vi "QuadRotor_Monitoring_LV2.vi"() -> ()   [LabVIEW 2015]
uses:
  <vilib>/Instr/_visa.llb/VISA Set IO Buffer Mask.ctl
  <vilib>/Instr/_visa.llb/VISA Configure Serial Port (Instr).vi
panel:
  out "MotorBackRf":dbl(slide) scale=1000.0..2000.0
  out "MotorBackLf":dbl(slide) scale=1000.0..2000.0
  out "MotorFrontRf":dbl(slide) scale=1000.0..2000.0
  out "MotorFrontLf":dbl(slide) scale=1000.0..2000.0
  in  "Lontitude_W3":i32=1005738310
  in  "Latitude_W3":i32=139458720
  in  "Lontitude_W2":i32=1005738310
  in  "Latitude_W2":i32=139458720
  in  "Lontitude_W1":i32=1005738310
  in  "Latitude_W1":i32=139458720
  in  "Lon_home":i32=1005748870
  in  "Lat_home":i32=139456050
  out "(GPS_numSat)":u16
  out "return count 2":u32
  out "Roob":i32
  out "Altitude_(Auto)":ext format="%#_3g"
  in  "Set_Altitude_(Auto)":dbl=2.5
  out "string":string
  out "Mode":ext format="%.2f"
  out "Altitude":dbl(slide) scale=0.0..20.0
  out "Altitude":ext format="%.2f"
  out "Yaw":dbl(knob) scale=-180.0..180.0
  out "Pitch":dbl(knob) scale=-90.0..90.0
  out "Roll":dbl(knob) scale=-90.0..90.0
  in  "Write to Quad":bool
  out "Header_58":u8
  out "GPS_Longtitude":ext format="%#.7f"
  out "Pitch":ext format="%.2f"
  out "Yaw":ext format="%.2f"
  out "GPS_Latitude":ext format="%#.7f"
  out "Roll":ext format="%.2f"
  out "return count":u32
  in  "stop":bool
  in  "VISA Serial Data":refnum<visa-resource-name>
  # "Quad Rotor Monitoring and Control with GPS Waypoint"
  # "Data Write to Autonomous Quad Rotor (LAT 9 Point), (LON 10 Point) with Google Map tracking Navigator"
  # "Ex  13.8591411 = 138591411 , 100.5231704 = 1005231704 Using in integer  I32"
  # "9 Point"
  # "10 Point"
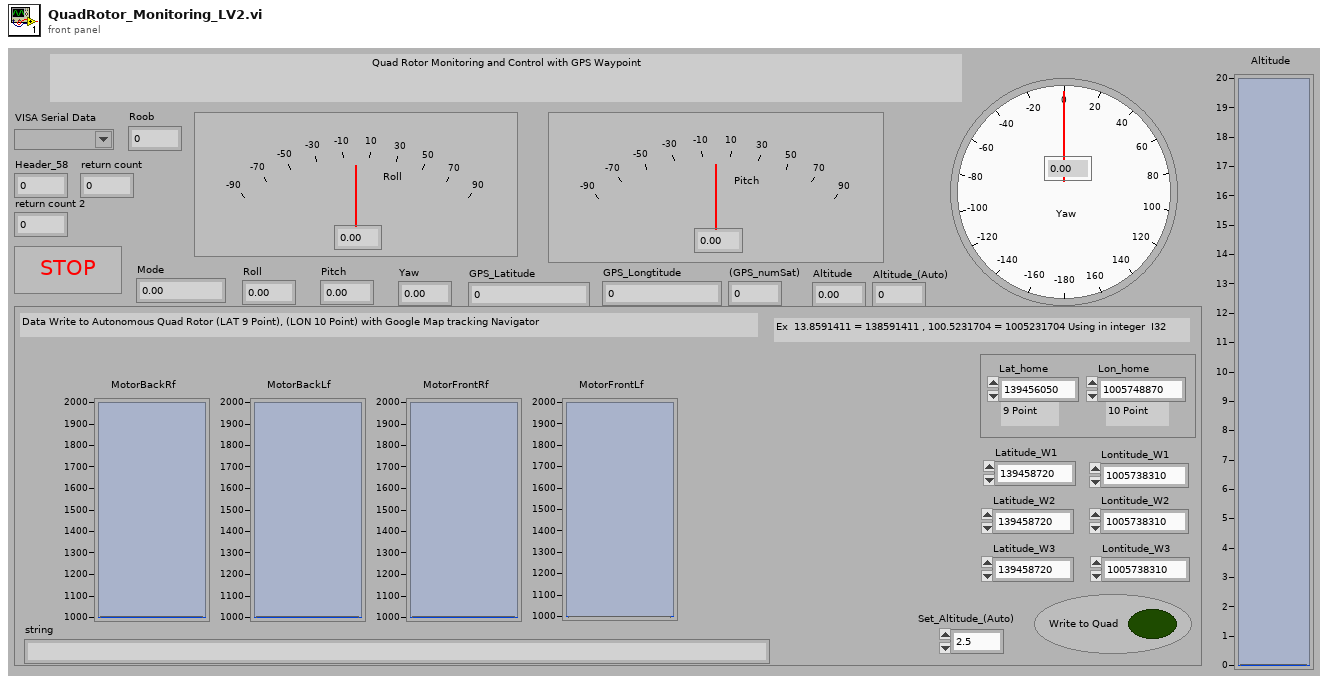
[diagram p1: front panel]
types:
  T1 = typedef "VISA Set IO Buffer Mask.ctl" = u16
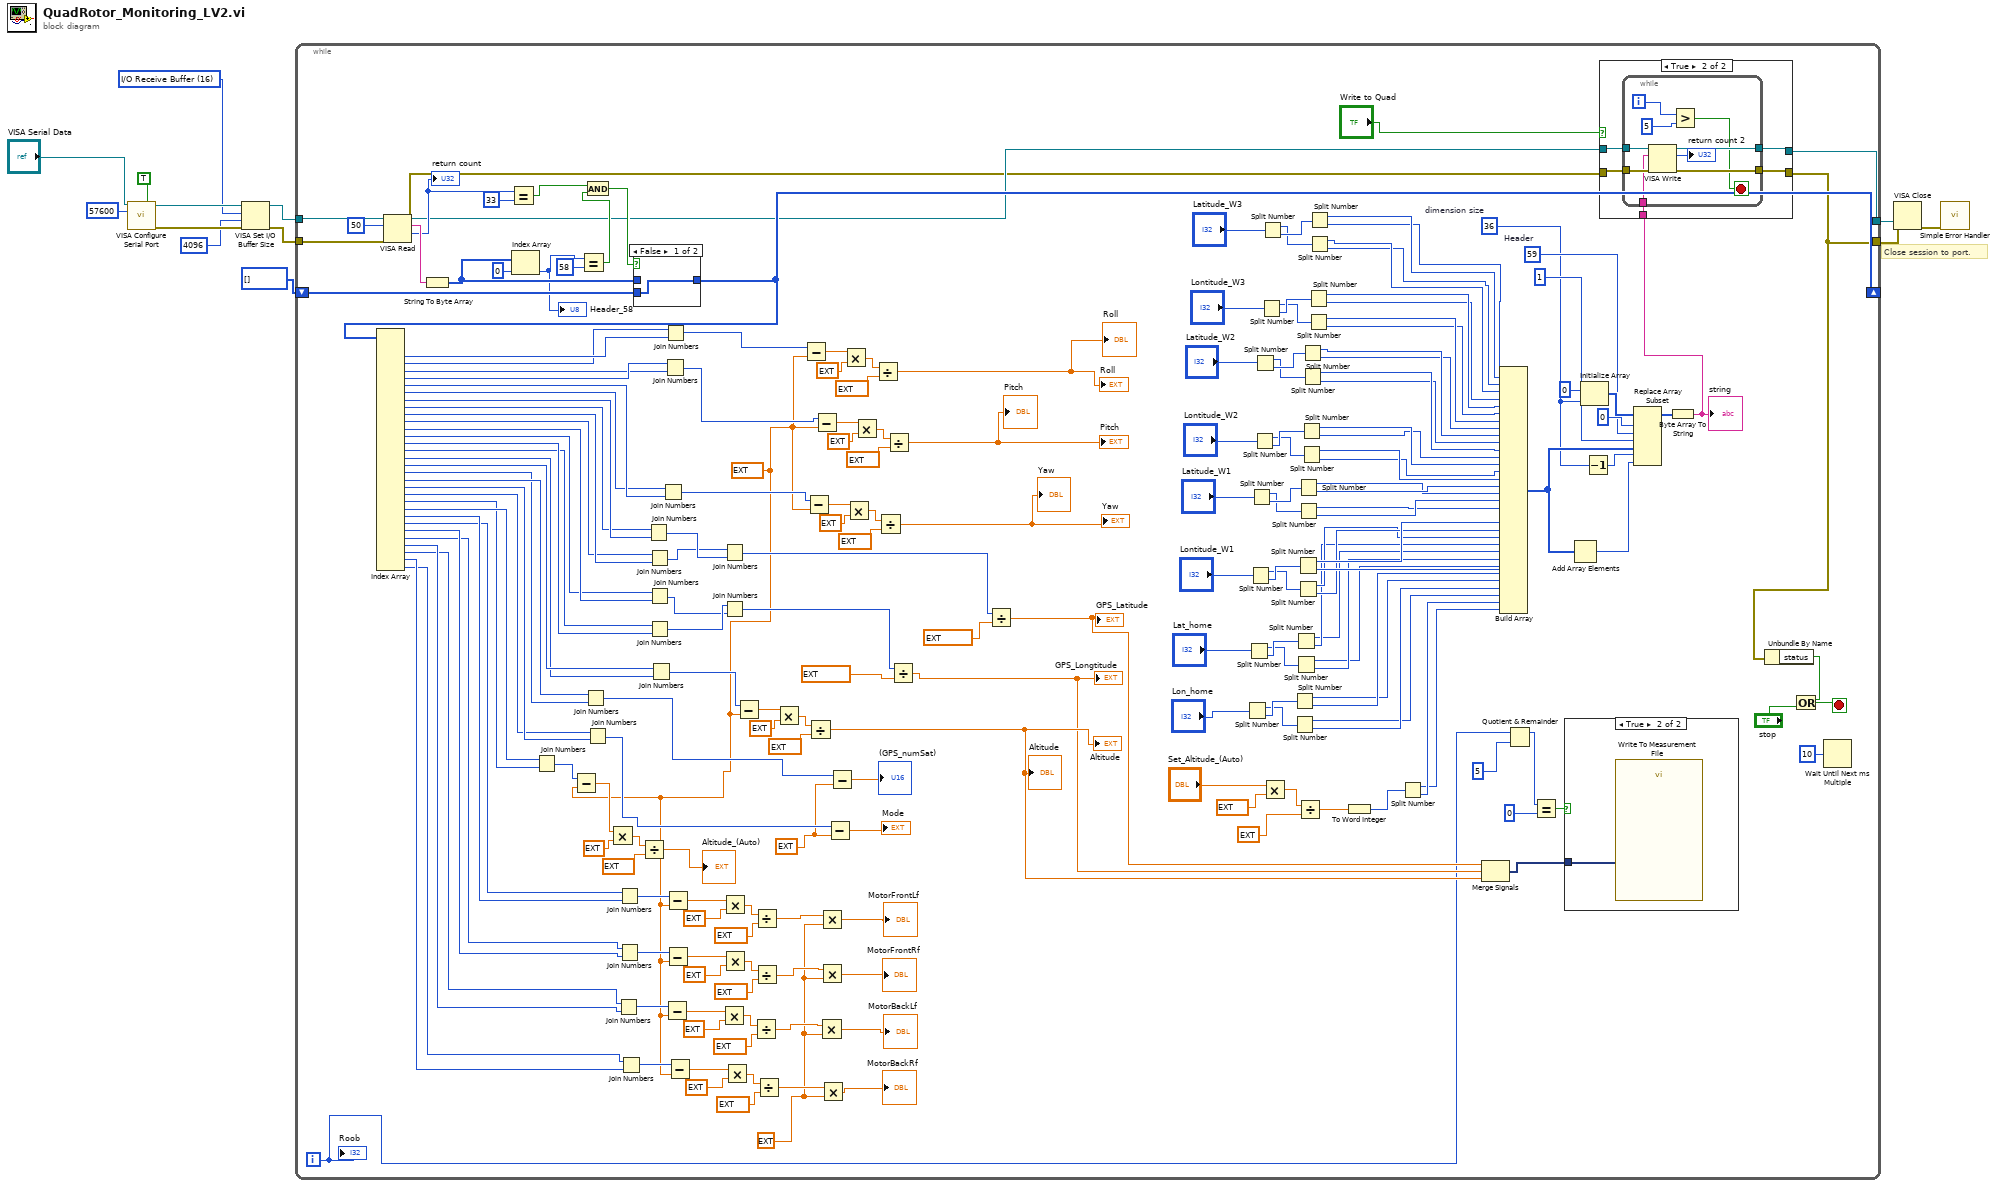
[diagram p0: block diagram]
diagram:
  w10 = T1 16 items=["I/O Receive Buffer"=16, "I/O Transmit Buffer"=32, "I/O Receive and Transmit Buffer"=48] ("Mask")
  # "Close session to port."
  n1 = call-poly "VISA Configure Serial Port"("VISA resource name"="VISA Serial Data", "Enable Termination\nChar (T)"=TRUE ("Enable Termination\nChar (T)"), "baud rate (9600)"=u32 57600) -> ("VISA resource name out"=w12:refnum<visa-resource-name>, "error out"=w11:errorcluster)  [unwired: 7 in, 4 out]
  n2 = VISA Set I/O Buffer Size(VISA resource name=w12, mask (16)=w10, size (4096)=u32 4096, error in (no error)=w11) -> (VISA resource name out=w8:refnum<visa-resource-name>, error out=w6:errorcluster)
  n3 = while {
    tunnel: [w179] -> w7
    tunnel: w8 -> [w220]
    tunnel: [w178] -> w5
    tunnel: w6 -> [w219]
    shift-right: [w189] -> _
    shift-left: u8[] [] ("unsigned byte array") -> [w190]
    i -> [w83]
    stop <- w223 stop-if-true
    w14 = ext 10.0 ("y")
    w98 = 36  # dimension size
    w146 = u8 59  # Header
    w90 = ext 255.0 ("y")
    w27 = ext 32767.0 ("y")
    n4 = VISA Read(VISA resource name=w220, byte count=u32 50, error in (no error)=w219) -> (VISA resource name out=w181:refnum<visa-resource-name>, read buffer=w193:string, return count=w186:u32, error out=w180:errorcluster)
    "return count" <- w186
    n5 = String To Byte Array(string=w193) -> (unsigned byte array=w191:u8[])
    n6 = Equal?(x=w186, y=u32 33) -> (x = y?=w184:bool)
    n7 = Index Array(array=w191, index=0) -> (element=w183:u8)
    "Header_58" <- w183
    n8 = Equal?(x=w183, y=u8 58) -> (x = y?=w188:bool)
    n9 = And(x=w184, y=w188) -> (x .and. y?=w187:bool)
    n10 = case shown="False" w187 {
      tunnel: w191 -> [_ w242]
      tunnel: [w241 w242] -> w189
      tunnel: w190 -> [w241 _]
      frame False {
      }
      frame True {
      }
    }
    n11 = Index Array(array=w189) -> (element #2=w213:u8, element #3=w212:u8, element #4=w210:u8, element #5=w211:u8, element #6=w217:u8, element #7=w216:u8, element #8=w215:u8, element #9=w214:u8, element #10=w174:u8, element #11=w173:u8, element #12=w170:u8, element #13=w169:u8, element #14=w168:u8, element #15=w167:u8, element #16=w157:u8, element #17=w163:u8, element #18=w155:u8, element #19=w156:u8, element #20=w154:u8, element #21=w153:u8, element #22=w109:u8, element #23=w110:u8, element #24=w31:u8, element #25=w30:u8, element #26=w29:u8, element #27=w28:u8, element #28=w26:u8, element #29=w25:u8, element #30=w24:u8, element #31=w23:u8)  [unwired: 31 in, 1 out]
    n12 = Join Numbers(hi=w110, lo=w109) -> ((hi.lo)=w108:u16)
    n13 = Subtract(x=w108, y=w27) -> (x-y=w104:ext)
    n14 = Join Numbers(hi=w156, lo=w155) -> ((hi.lo)=w89:u16)
    n15 = Join Numbers(hi=w153, lo=w154) -> ((hi.lo)=w93:u16)
    n16 = Multiply(x=w104, y=ext 100.0) -> (x*y=w106:ext)
    n17 = Join Numbers(hi=w25, lo=w26) -> ((hi.lo)=w37:u16)
    n18 = Join Numbers(hi=w30, lo=w31) -> ((hi.lo)=w47:u16)
    n19 = Join Numbers(hi=w28, lo=w29) -> ((hi.lo)=w42:u16)
    n20 = Join Numbers(hi=w23, lo=w24) -> ((hi.lo)=w32:u16)
    n21 = Divide(x=w106, y=ext 32767.0) -> (x/y=→"Altitude_(Auto)":ext)
    n22 = Join Numbers(hi=w214, lo=w215) -> ((hi.lo)=w172:u16)
    n23 = Join Numbers(hi=w173, lo=w174) -> ((hi.lo)=w171:u16)
    n24 = Join Numbers(hi=w169, lo=w170) -> ((hi.lo)=w151:u16)
    n25 = Join Numbers(hi=w167, lo=w168) -> ((hi.lo)=w152:u16)
    n26 = Join Numbers(hi=w163, lo=w157) -> ((hi.lo)=w158:u16)
    n27 = Join Numbers(hi=w216, lo=w217) -> ((hi.lo)=w199:u16)
    n28 = Join Numbers(hi=w211, lo=w210) -> ((hi.lo)=w194:u16)
    n29 = Join Numbers(hi=w212, lo=w213) -> ((hi.lo)=w208:u16)
    n30 = Subtract(x=w37, y=w27) -> (x-y=w40:ext)
    n31 = Subtract(x=w47, y=w27) -> (x-y=w50:ext)
    n32 = Subtract(x=w42, y=w27) -> (x-y=w45:ext)
    n33 = Subtract(x=w32, y=w27) -> (x-y=w35:ext)
    n34 = Multiply(x=w40, y=ext 185.0) -> (x*y=w41:ext)
    n35 = Join Numbers(hi=w171, lo=w172) -> ((hi.lo)=w176:u32)
    n36 = Join Numbers(hi=w152, lo=w151) -> ((hi.lo)=w166:u32)
    n37 = Multiply(x=w50, y=ext 185.0) -> (x*y=w51:ext)
    n38 = Multiply(x=w45, y=ext 185.0) -> (x*y=w46:ext)
    n39 = Multiply(x=w35, y=ext 185.0) -> (x*y=w36:ext)
    n40 = Subtract(x=w158, y=w27) -> (x-y=w162:ext)
    n41 = Divide(x=w41, y=ext 32767.0) -> (x/y=w17:ext)
    n42 = Divide(x=w51, y=ext 32767.0) -> (x/y=w15:ext)
    n43 = Divide(x=w46, y=ext 32767.0) -> (x/y=w16:ext)
    n44 = Divide(x=w36, y=ext 32767.0) -> (x/y=w22:ext)
    n45 = Multiply(x=w162, y=ext 100.0) -> (x*y=w160:ext)
    n46 = Subtract(x=w208, y=w27) -> (x-y=w207:ext)
    n47 = Subtract(x=w199, y=w27) -> (x-y=w203:ext)
    n48 = Divide(x=w160, y=ext 32767.0) -> (x/y=w88:ext)
    "Altitude" <- w88
    "Altitude" <- w88
    n49 = Subtract(x=w194, y=w27) -> (x-y=w198:ext)
    n50 = Multiply(x=w17, y=w14) -> (x*y=→"MotorBackLf":ext)
    n51 = Multiply(x=w15, y=w14) -> (x*y=→"MotorFrontLf":ext)
    n52 = Multiply(x=w16, y=w14) -> (x*y=→"MotorFrontRf":ext)
    n53 = Multiply(x=w22, y=w14) -> (x*y=→"MotorBackRf":ext)
    n54 = Subtract(x=w93, y=w90) -> (x-y=→"Mode":ext)
    n55 = Subtract(x=w89, y=w90) -> (x-y=→"(GPS_numSat)":ext)
    n56 = Multiply(x=w207, y=ext 180.0) -> (x*y=w205:ext)
    n57 = Multiply(x=w203, y=ext 180.0) -> (x*y=w201:ext)
    n58 = Multiply(x=w198, y=ext 180.0) -> (x*y=w196:ext)
    n59 = Divide(x=w205, y=ext 32767.0) -> (x/y=→"Roll" →"Roll":ext)
    n60 = Divide(x=w201, y=ext 32767.0) -> (x/y=→"Yaw" →"Yaw":ext)
    n61 = Divide(x=w196, y=ext 32767.0) -> (x/y=→"Pitch" →"Pitch":ext)
    n62 = Divide(x=w166, y=ext 10000000.0) -> (x/y=w87:ext)
    "GPS_Longtitude" <- w87
    n63 = Divide(x=w176, y=ext 10000000.0) -> (x/y=w86:ext)
    "GPS_Latitude" <- w86
    n64 = Split Number(x="Lon_home") -> (hi(x)=w139:u16, lo(x)=w140:u16)
    n65 = Split Number(x="Lat_home") -> (hi(x)=w141:u16, lo(x)=w142:u16)
    n66 = Split Number(x="Lontitude_W1") -> (hi(x)=w143:u16, lo(x)=w144:u16)
    n67 = Split Number(x="Latitude_W1") -> (hi(x)=w121:u16, lo(x)=w122:u16)
    n68 = Split Number(x="Lontitude_W2") -> (hi(x)=w78:u16, lo(x)=w79:u16)
    n69 = Split Number(x="Latitude_W2") -> (hi(x)=w76:u16, lo(x)=w77:u16)
    n70 = Split Number(x="Lontitude_W3") -> (hi(x)=w72:u16, lo(x)=w73:u16)
    n71 = Split Number(x="Latitude_W3") -> (hi(x)=w70:u16, lo(x)=w71:u16)
    n72 = Multiply(x="Set_Altitude_(Auto)", y=ext 32767.0) -> (x*y=w113:ext)
    n73 = Split Number(x=w140) -> (hi(x)=w125:u8, lo(x)=w126:u8)
    n74 = Split Number(x=w139) -> (hi(x)=w123:u8, lo(x)=w124:u8)
    n75 = Split Number(x=w142) -> (hi(x)=w129:u8, lo(x)=w130:u8)
    n76 = Split Number(x=w141) -> (hi(x)=w127:u8, lo(x)=w128:u8)
    n77 = Split Number(x=w144) -> (hi(x)=w133:u8, lo(x)=w134:u8)
    n78 = Split Number(x=w143) -> (hi(x)=w131:u8, lo(x)=w132:u8)
    n79 = Split Number(x=w122) -> (hi(x)=w137:u8, lo(x)=w138:u8)
    n80 = Split Number(x=w121) -> (hi(x)=w135:u8, lo(x)=w136:u8)
    n81 = Divide(x=w113, y=ext 100.0) -> (x/y=w111:ext)
    n82 = Split Number(x=w79) -> (hi(x)=w65:u8, lo(x)=w64:u8)
    n83 = Split Number(x=w78) -> (hi(x)=w67:u8, lo(x)=w66:u8)
    n84 = Split Number(x=w77) -> (hi(x)=w61:u8, lo(x)=w60:u8)
    n85 = Split Number(x=w76) -> (hi(x)=w63:u8, lo(x)=w62:u8)
    n86 = Split Number(x=w73) -> (hi(x)=w57:u8, lo(x)=w56:u8)
    n87 = Split Number(x=w72) -> (hi(x)=w59:u8, lo(x)=w58:u8)
    n88 = Split Number(x=w71) -> (hi(x)=w53:u8, lo(x)=w52:u8)
    n89 = Split Number(x=w70) -> (hi(x)=w55:u8, lo(x)=w54:u8)
    n90 = To Word Integer(number=w111) -> (16bit integer=w114:i16)
    n91 = Split Number(x=w114) -> (hi(x)=w115:u8, lo(x)=w116:u8)
    n92 = Merge Signals(w86, w87, w88) -> (w85:dynamicdata)
    n93 = Build Array(w52, w53, w54, w55, w56, w57, w58, w59, w60, w61, w62, w63, w64, w65, w66, w67, w138, w137, w136, w135, w134, w133, w132, w131, w130, w129, w128, w127, w126, w125, w124, w123, w116, w115) -> (w101:u8[])
    n94 = Quotient & Remainder(x=w83, y=u32 5) -> (x-y*floor(x/y)=w80:u32)  [unwired: 1 out]
    n95 = Equal?(x=w80, y=u32 0) -> (x = y?=w82:bool)
    n96 = case shown="True" w82 {
      tunnel: w85 -> [_ w224]
      frame False {
      }
      frame True {
        n97 = call "Write To Measurement File"("Signals"=w224) -> ()  [unwired: 16 in, 3 out]
      }
    }
    n98 = Add Array Elements(numeric array=w101) -> (sum=w100:u8)
    n99 = Initialize Array(u8 0, w98) -> (w150:u8[])
    n100 = Decrement(x=w98) -> (x-1=w99:i32)
    n101 = Replace Array Subset(array=w150, new element #1=w146, index #1=0 ("index"), new element #2=w101, index #2=1 ("index"), new element #3=w100, index #3=w99) -> (w145:u8[])
    n102 = Byte Array To String(unsigned byte array=w145) -> (string=w120:string)
    "string" <- w120
    n103 = case shown="True" "Write to Quad" {
      tunnel: w181 -> [w225 w231]
      tunnel: w180 -> [w226 w228]
      tunnel: [w225 w230] -> w179
      tunnel: [w226 w229] -> w178
      tunnel: w120 -> [_ w227]
      frame False {
      }
      frame True {
        n104 = while {
          tunnel: w231 -> [w240]
          tunnel: [w239] -> w230
          tunnel: [w238] -> w229
          tunnel: w228 -> [w237]
          tunnel: w227 -> [w236]
          i -> [w234]
          stop <- w232 stop-if-true
          n105 = VISA Write(VISA resource name=w240, write buffer=w236, error in (no error)=w237) -> (VISA resource name out=w239:refnum<visa-resource-name>, return count=→"return count 2":u32, error out=w238:errorcluster)
          n106 = Greater?(x=w234, y=5) -> (0:w232:bool)
        }
      }
    }
    n107 = Unbundle By Name(w178) -> ("status"=w221:bool)
    n108 = Or(x=w221, y="stop") -> (x .or. y?=w223:bool)
    n109 = Wait Until Next ms Multiple(millisecond multiple=u32 10) -> ()  [unwired: 1 out]
    "Roob" <- w83
  }
  n110 = VISA Close(VISA resource name=w7, error in (no error)=w5) -> (error out=w9:errorcluster)
  n111 = call <vilib>:"Simple Error Handler.vi"("error in (no error)"=w9) -> ()  [unwired: 1 in, 8 out]
